vi "AM_Freq_Resp.vi"() -> ()   [LabVIEW 2018]
doc: "Use Arduino Micro and SparkFun MiniGen to measure Frequency Response of a Load\n\nR. Sheehan 18 - 11 - 2020"
uses:
  <vilib>/Instr/_visa.llb/VISA Configure Serial Port (Instr).vi
panel:
  in  "Tab Control":T1(tab)
  in  "Addr":refnum<visa-resource-name>
  in  "Open Comms":bool
  out "Addr 2":refnum<visa-resource-name>
  out "Open":bool
  in  "Write f":bool
  in  "Frequency / Hz":dbl min=0.0 max=3.3
  in  "Delay (ms)":u32
  out "Cmd":string
  in  "Nreads":i32
  in  "Read":bool
  out "Meas / V":dbl[](array[numeric])
  out "Err / V":dbl[](array[numeric])
  out "Buffer Size":i32
  out "Buffer Data 2":string[](array[string])
  in  "fdelta / kHz":dbl
  in  "fhigh / kHz":dbl
  in  "flow / kHz":dbl
  in  "Sweep Meas.":bool
  out "XY Graph":cluster{dbl[], dbl[]}(graph)
  out "error out":errorcluster
  in  "Stop":bool
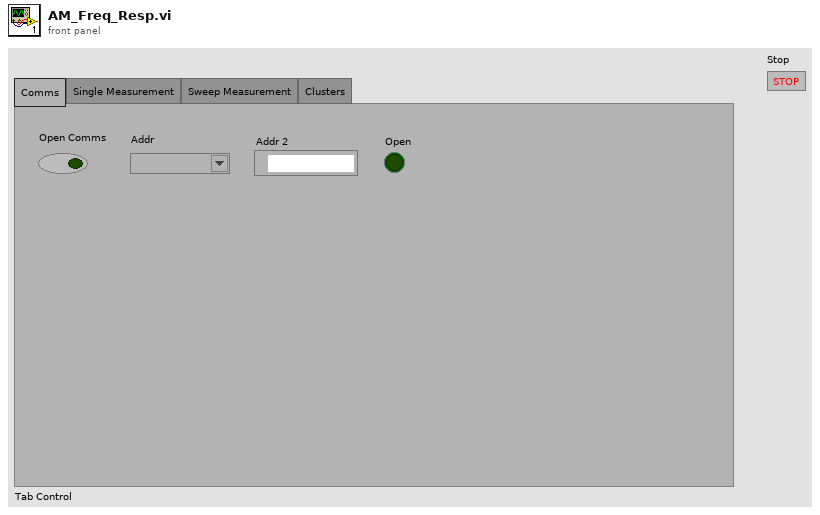
[diagram p1: front panel]
types:
  T1 = enum32{"Comms", "Single Measurement", "Sweep Measurement", "Clusters"}
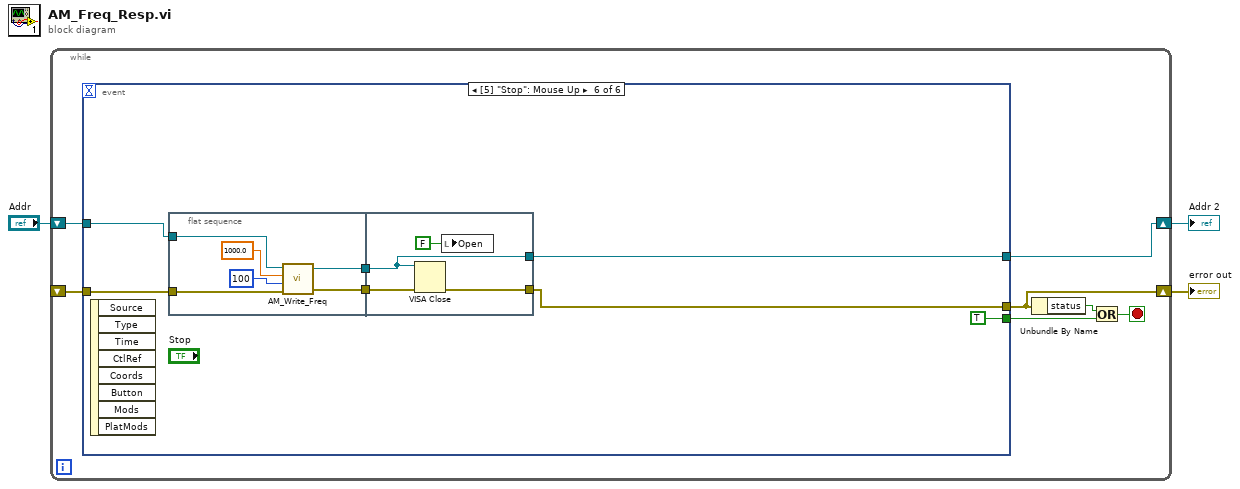
[diagram p0: block diagram]
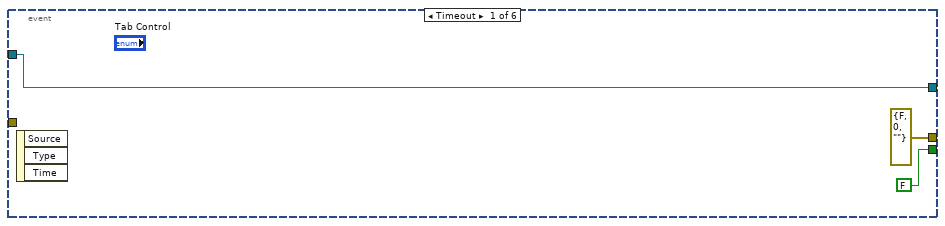
[diagram p2: hidden frame]
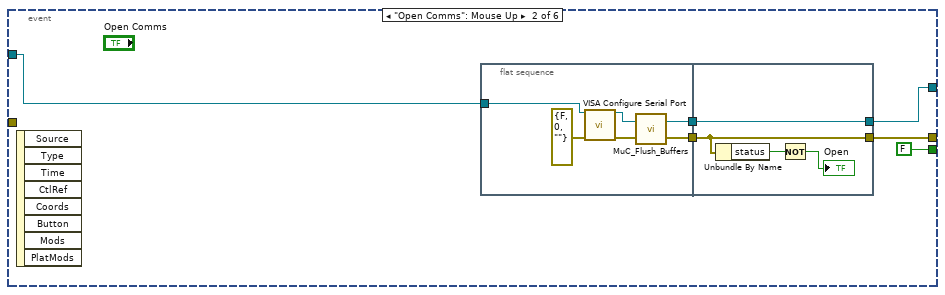
[diagram p3: hidden frame]
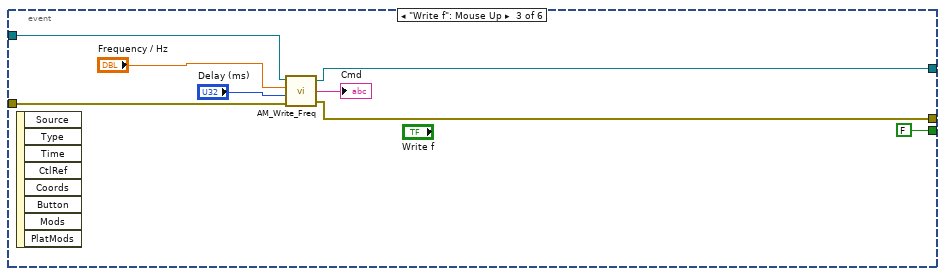
[diagram p4: hidden frame]
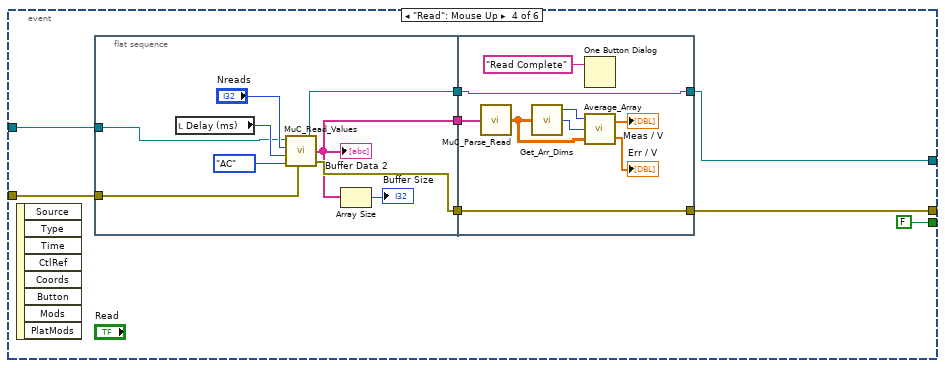
[diagram p5: hidden frame]
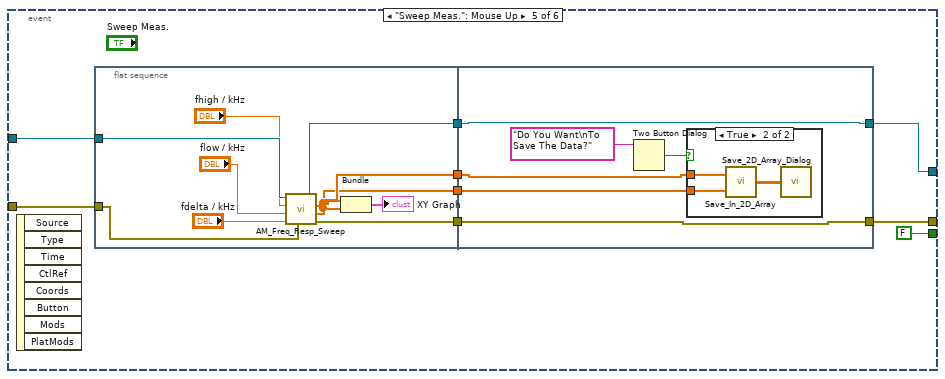
[diagram p6: hidden frame]
diagram:
  n1 = while {
    shift-right: [w9] -> w2
    shift-left: "Addr" -> [w10]
    shift-right: [w8] -> w1
    shift-left: _ -> [w7]
    stop <- w5 stop-if-true
    n2 = event shown="[5] \"Stop\": Mouse Up" {
      selector: _ -> [_ _ _ _ _ _]
      dyn-events: _ -> [_ _ _ _ _ _]
      timeout: _ -> [_ _ _ _ _ _]
      tunnel: w10 -> [w11 w19 w36 w44 w70 w95]
      tunnel: [w11 w17 w33 w42 w69 w93] -> w9
      tunnel: [errorcluster {"status"=FALSE, "code"=0, "source"=""} ("error in (no error)") w14 w32 w41 w68 w97] -> w8
      tunnel: w7 -> [_ _ w35 w43 w71 w96]
      tunnel: [FALSE FALSE FALSE FALSE FALSE TRUE] -> w4
      event Timeout {
        n3 = event-data() -> ()  [unwired: 1 in, 3 out]
      }
      event "Open Comms": Mouse Up {
        n4 = event-data() -> ()  [unwired: 1 in, 8 out]
        n5 = flat-sequence {
          tunnel: w19 -> [w24]
          tunnel: [w22] -> w16
          tunnel: [w20] -> w15
          tunnel: [w29] -> w17
          tunnel: w16 -> [w29]
          tunnel: w15 -> [w28]
          tunnel: [w28] -> w14
          frame #0 {
            n6 = call-poly "VISA Configure Serial Port"("VISA resource name"=w24, "error in (no error)"=errorcluster {"status"=FALSE, "code"=0, "source"=""}) -> ("VISA resource name out"=w23:refnum<visa-resource-name>, "error out"=w21:errorcluster)  [unwired: 7 in, 5 out]
            n7 = call "MuC_Flush_Buffers.vi"("error in (no error)"=w21, "VISA resource name"=w23) -> ("error out"=w20:errorcluster, "VISA resource name 2"=w22:refnum<visa-resource-name>)
          }
          frame #1 {
            n8 = Unbundle By Name(w28) -> ("status"=w26:bool)
            n9 = Not(x=w26) -> (.not. x?=→"Open":bool)
          }
        }
      }
      event "Write f": Mouse Up {
        n10 = event-data() -> ()  [unwired: 1 in, 8 out]
        n11 = call "AM_Write_Freq.vi"("error in (no error)"=w35, "Delay / ms"="Delay (ms)", "f / Hz"="Frequency / Hz", "VISA resource name"=w36) -> ("error out"=w32:errorcluster, "Cmd"=→"Cmd":string, "VISA resource name 2"=w33:refnum<visa-resource-name>)
      }
      event "Read": Mouse Up {
        n12 = event-data() -> ()  [unwired: 1 in, 8 out]
        n13 = flat-sequence {
          tunnel: w44 -> [w49]
          tunnel: w43 -> [w48]
          tunnel: [w54] -> w40
          tunnel: [w53] -> w39
          tunnel: [w47] -> w38
          tunnel: [w62] -> w41
          tunnel: [w63] -> w42
          tunnel: w40 -> [w63]
          tunnel: w39 -> [w62]
          tunnel: w38 -> [w55]
          frame #0 {
            n14 = local read "Delay (ms)"() -> (w52:u32)
            n15 = call "MuC_Read_Values.vi"("VISA resource name"=w49, "Nreads"="Nreads", "Delay (ms)"=w52, "Read Type"=enum16{"DC", "AC"}."AC", "error in (no error)"=w48) -> ("VISA resource name 2"=w54:refnum<visa-resource-name>, "Buffer Data"=w47:string[], "error out"=w53:errorcluster)
            "Buffer Data 2" <- w47
            n16 = Array Size(array=w47) -> (size(s)=→"Buffer Size":i32)
          }
          frame #1 {
            n17 = call "MuC_Parse_Read.vi"("Buffer Data"=w55) -> ("Data"=w58:dbl[][])
            n18 = call "Get_Arr_Dims.vi"("Data"=w58) -> ("N Rows"=w57:i32, "N Cols"=w56:i32)  [unwired: 1 out]
            n19 = One Button Dialog(message="Read Complete") -> ()  [unwired: 1 in, 1 out]
            n20 = call "Average_Array.vi"("Array"=w58, "Ncolumns"=w56, "Nrows"=w57) -> ("Max-Min"=→"Err / V":dbl[], "Average"=→"Meas / V":dbl[])
          }
        }
      }
      event "Sweep Meas.": Mouse Up {
        n21 = event-data() -> ()  [unwired: 1 in, 8 out]
        n22 = flat-sequence {
          tunnel: w71 -> [w82]
          tunnel: w70 -> [w81]
          tunnel: [w80] -> w67
          tunnel: [w79] -> w66
          tunnel: [w74] -> w65
          tunnel: [w73] -> w64
          tunnel: [w87] -> w68
          tunnel: [w88] -> w69
          tunnel: w67 -> [w88]
          tunnel: w66 -> [w87]
          tunnel: w65 -> [w84]
          tunnel: w64 -> [w83]
          frame #0 {
            n23 = call "AM_Freq_Resp_Sweep.vi"("error in"=w82, "fdelta / kHz"="fdelta / kHz", "flow / kHz"="flow / kHz", "fhigh / kHz"="fhigh / kHz", "VISA resource name 2"=w81) -> ("error out"=w79:errorcluster, "Rdata"=w73:dbl[], "Fdata"=w74:dbl[], "VISA resource name 3"=w80:refnum<visa-resource-name>)
            n24 = Bundle("Fdata"=w74, "Rdata"=w73) -> (→"XY Graph":cluster{"Fdata":dbl[], "Rdata":dbl[]})  [unwired: 1 in]
          }
          frame #1 {
            n25 = Two Button Dialog(message="Do You Want\nTo Save The Data?") -> (T button?=w85:bool)  [unwired: 2 in]
            n26 = case shown="True" w85 {
              tunnel: w84 -> [_ w91]
              tunnel: w83 -> [_ w90]
              frame False {
              }
              frame True {
                n27 = call "Save_In_2D_Array.vi"("Vert"=w90, "Horz"=w91) -> ("Array"=w89:dbl[][])
                n28 = call "Save_2D_Array_Dialog.vi"("2D data"=w89) -> ()
              }
            }
          }
        }
      }
      event "Stop": Mouse Up {
        n29 = event-data() -> ()  [unwired: 1 in, 8 out]
        n30 = flat-sequence {
          tunnel: w96 -> [w101]
          tunnel: w95 -> [w104]
          tunnel: [w103] -> w94
          tunnel: [w102] -> w92
          tunnel: [w108] -> w97
          tunnel: w94 -> [w106]
          tunnel: [w106] -> w93
          tunnel: w92 -> [w105]
          frame #0 {
            n31 = call "AM_Write_Freq.vi"("error in (no error)"=w101, "Delay / ms"=u32 100, "f / Hz"=1000.0, "VISA resource name"=w104) -> ("error out"=w102:errorcluster, "VISA resource name 2"=w103:refnum<visa-resource-name>)  [unwired: 1 out]
          }
          frame #1 {
            n32 = VISA Close(VISA resource name=w106, error in (no error)=w105) -> (error out=w108:errorcluster)
            n33 = local write "Open"(FALSE) -> ()
          }
        }
      }
    }
    n34 = Unbundle By Name(w8) -> ("status"=w6:bool)
    n35 = Or(x=w6, y=w4) -> (x .or. y?=w5:bool)
  }
  "Addr 2" <- w2
  "error out" <- w1
